vi "Actor Core.vi"(8 "error in":errorcluster, 11 "RDS Test Child in":refnum<class "RDS Test Child.lvclass">) -> (0 "error out":errorcluster, 3 "Actor out":refnum<class "Actor.lvclass">)   [LabVIEW 2015, in "RDS Test Child.lvlib" / "RDS Test Child.lvclass"]
doc: "(<B>Filename</B>: Actor Framework.lvlib:Actor.lvclass:Actor Core.vi)\n\nReceives messages to the actor, reacts to them, and initiates any error handling that may shut the actor down.\n\nDescendant classes may override this VI to append parallel tasks for the actor to complete while it handles messages. Overrides use the Call Parent Method node."
uses:
  RDS Test Child.lvclass
  RDS Parent Actor/RDS Parent Actor/RDS Parent Actor.lvclass
  <vilib>/ActorFramework/Actor/Actor.lvclass
  <vilib>/ActorFramework/Stop Msg/Stop Msg.lvclass
  Libraries/RDS Framework/RDS Message Class/RDS Message.lvclass
  Libraries/RDS Framework/RDS Message ID.ctl
  Libraries/RDS Child Messages/RDS Child Messages.lvlib
  Libraries/RDS Child Messages/String Message/String Message.lvclass
  Libraries/RDS Framework/RDS Message Class/AIP Command.lvclass
  Libraries/RDS Framework/RDS Message Class/AIP Command Control.ctl
  Libraries/RDS Child Messages/MCB/MCB Command Message/MCB Command.lvclass
  Libraries/RDS Child Messages/MCB/MCB Channel.ctl
  Libraries/3rd Party/Artificial Horizon/lv-attitudecontrol.lvlib
  Libraries/RDS Child Messages/Helm/Helm Limiter Message/Helm Limiter Msg.lvclass
  Libraries/RDS Child Messages/Helm/Heading Command/Heading Command Msg.lvclass
  Libraries/RDS Child Messages/Helm/Steering Command/Steering Command.lvclass
  Libraries/RDS Child Messages/Controller Message/Controller Message.lvclass
  Libraries/RDS Child Messages/Controller Message/Controller Message Type.ctl
  RDS Controller Actor/RDS Controller Actor/Controller.ctl
  RDS Controller Actor/RDS Controller Actor/RDS Controller Actor.lvlib
  RDS State Tracker/RDS State/RDS State.lvclass
  Libraries/RDS Child Messages/Depth Data Message/Depth Data Message.lvclass
  Libraries/RDS Child Messages/AIP Set Min Depth Message/AIP Set Min Depth Message.lvclass
  Compass Instrument/Compass Instrument.lvlib
  RDS Mission Controller Actor/RDS Mission Controller Actor.lvlib
  RDS Mission Controller Actor/MissionOp.ctl
  Libraries/RDS Child Messages/PID Gains/PID Gains Set Message.lvclass
  Libraries/RDS Instruments/AIP/AIP States.ctl
  Libraries/RDS Instruments/RDS Instrument Library.lvlib
  Libraries/RDS Instruments/AIP/AIP Status.ctl
  Libraries/3rd Party/NMEA_GPS/NMEA_LatitudeDirection.ctl
  Libraries/3rd Party/NMEA_GPS/NMEA.lvlib
  Libraries/3rd Party/NMEA_GPS/NMEA_LongitudeDirection.ctl
  Libraries/3rd Party/NMEA_GPS/NMEA_GPRMC-data.ctl
  Libraries/RDS Child Messages/MCB/MCB Motor Status.ctl
  Libraries/RDS Instruments/Compass/Compass Data.ctl
  RDS Helm Actor/RDS Helm Actor/Helm State.ctl
  RDS Helm Actor/RDS Helm Actor.lvlib
  Libraries/RDS Child Messages/Helm/Heading Command/Heading Command Cntrl.ctl
  Libraries/RDS Child Messages/Helm/Steering Command/Steering Command Cntrl.ctl
  Libraries/RDS Child Messages/PID Gains/PID Gains Control.ctl
  Libraries/RDS Child Messages/Helm/Helm Status Message/Helm Status Control.ctl
  Libraries/GUI/Throttles.ctl
  Libraries/Geo/RDS Libraries.lvlib
  Libraries/RDS Instruments/Battery/Battery Data.ctl
  Libraries/RDS Child Messages/Battery Data/Battery Status.ctl
  Libraries/RDS Child Messages/Depth Data Message/Depth Data.ctl
  RDS Mission Controller Actor/Mission Controller Navigation State.ctl
  Libraries/RDS Child Messages/Mission Messages/Mission Controller State Control.ctl
  Libraries/RDS Child Messages/Mission Messages/Mission Controller State Message.lvclass
  RDS Mission Controller Actor/Mission Controller Settings.ctl
panel:
  in  "Tab Control":T1(tab)
  out "Depth Time":timestamp
  in  "stop":bool
  out "$GPRMC Msg":T2={"TimeStamp"=timestamp(0 s since 1904-01-01), "Validity"=FALSE, "Latitude"=0.0, "Latitude-Direction"=enum."North", "Longitude"=0.0, "Longitude-Direction"=enum."East", "Speed in knots"=0.0, "True course"=0.0, "Date Stamp"=timestamp(0 s since 1904-01-01), "Magnetic Variation (East/West)"=0.0, "GPS Latitude"=0.0, "GPS Longitude"=0.0} {"GPS Longitude" format="%.6f"; "GPS Latitude" format="%.6f"; "Magnetic Variation (East/West)" format="%.02f [deg]"; "Date Stamp" format="%<%x>T"; "True course" format="%.02f [deg]"; "Speed in knots" format="%.02f [kts]"; "Longitude" format="%0.4f [long]"; "Latitude" format="%.04f [lat]"; "TimeStamp" format="%<%.2X>T"}
  in  "Port Throttle":i16
  in  "STBD Throttle":i16
  in  "Btn Port Throttle":bool
  in  "Btn STBD Throttle":bool
  out "Port Motor 2":T5
  out "STBD Motor 2":T5
  out "Compass Data":T6
  in  "Attitude Indicator":refnum<vi>(3d-picture)
  out "Depth":dbl
  out "Water Temp":dbl
  in  "btn_shutdown":bool
  in  "rckr_shutdown_safety":bool
  out "Battery Pack Time":timestamp
  out "GPS Frame Time":timestamp
  out "Compass Frame Time":timestamp
  out "Port Motor Time":timestamp
  out "STBD Motor Time":timestamp
  in  "AIP Stop":bool
  in  "AIP Stow":bool
  in  "AIP Deploy":bool
  out "AIP Status Time Stamp":timestamp
  out "AIP Status":T7
  out "Current Chart":dbl(graph)
  out "Battery Pack Info":T9
  in  "btn_gains set":bool
  in  "Gains":T11 {"D (Td)" format="%#_9f"; "I (Ti)" format="%#_9f"; "P (Kc)" format="%#.9f"}
  in  "Throttles":T12 {"STBD" scale=-1000.0..1000.0; "Port" scale=-1000.0..1000.0}
  in  "Steering Command":T13
  in  "Heading Command":T14
  in  "btn_limiter_set":bool
  in  "Limter":dbl(slide) min=0.0 max=100.0 scale=0.0..100.0
  out "Helm Status":T15 {"Gains"."D (Td)" format="%#_9f"; "Gains"."I (Ti)" format="%#_9f"; "Gains"."P (Kc)" format="%#.9f"}
  out "Rudder Chart":dbl(graph)
  out "PV and S Chart":cluster{"initial PV":dbl, "SP:":dbl}(graph)
  out "Helm Status Time":timestamp
  in  "btn_heading_command":bool
  in  "btn_steering_command":bool
  out "Message time":dbl
  in  "btn_set_mag_dev":bool
  in  "Compass Mag Dev":dbl
  in  "btn_set_aip_min_depth":bool
  in  "AIP Min Depth":dbl
  in  "btn_sim_depth_data":bool
  in  "Depth Data":T17
  in  "btn_shore_remote_ReqControl":bool
  in  "btn_shore_remote_Relinquish":bool
  in  "btn_local_remote_Relinquish":bool
  in  "btn_local_remote_ReqControl":bool
  in  "Send Msg":bool
  out "String":string
  in  "Send string":bool
  in  "String 2":string
  in  "btn_open_mission":bool
  in  "btn_save_mission":bool
  out "XY Graph":T18(graph)
  in  "btn_send settings":bool
  in  "btn_set_op_run":bool
  in  "btn_upload_mission":bool
  in  "Test Mission":T19[](array[typedef]) {"GPS Longitude" format="%.6g"; "GPS Latitude" format="%.6g"}
  out "Mission Controller State":T20 {"Mission"."GPS Longitude" format="%.6g"; "Mission"."GPS Latitude" format="%.6g"}
  in  "btn_mission_Relinquish":bool
  in  "btn_mission_ReqControl":bool
  in  "Mission Controller Settings":T22
  in  "MissionOp Index":i32
  in  "RDS State":refnum<class "RDS State.lvclass">
  out "State Sample Time":timestamp
  out "Controller State":T23
  out "Helm Status 2":T15 {"Gains"."D (Td)" format="%#_9f"; "Gains"."I (Ti)" format="%#_9f"; "Gains"."P (Kc)" format="%#.9f"}
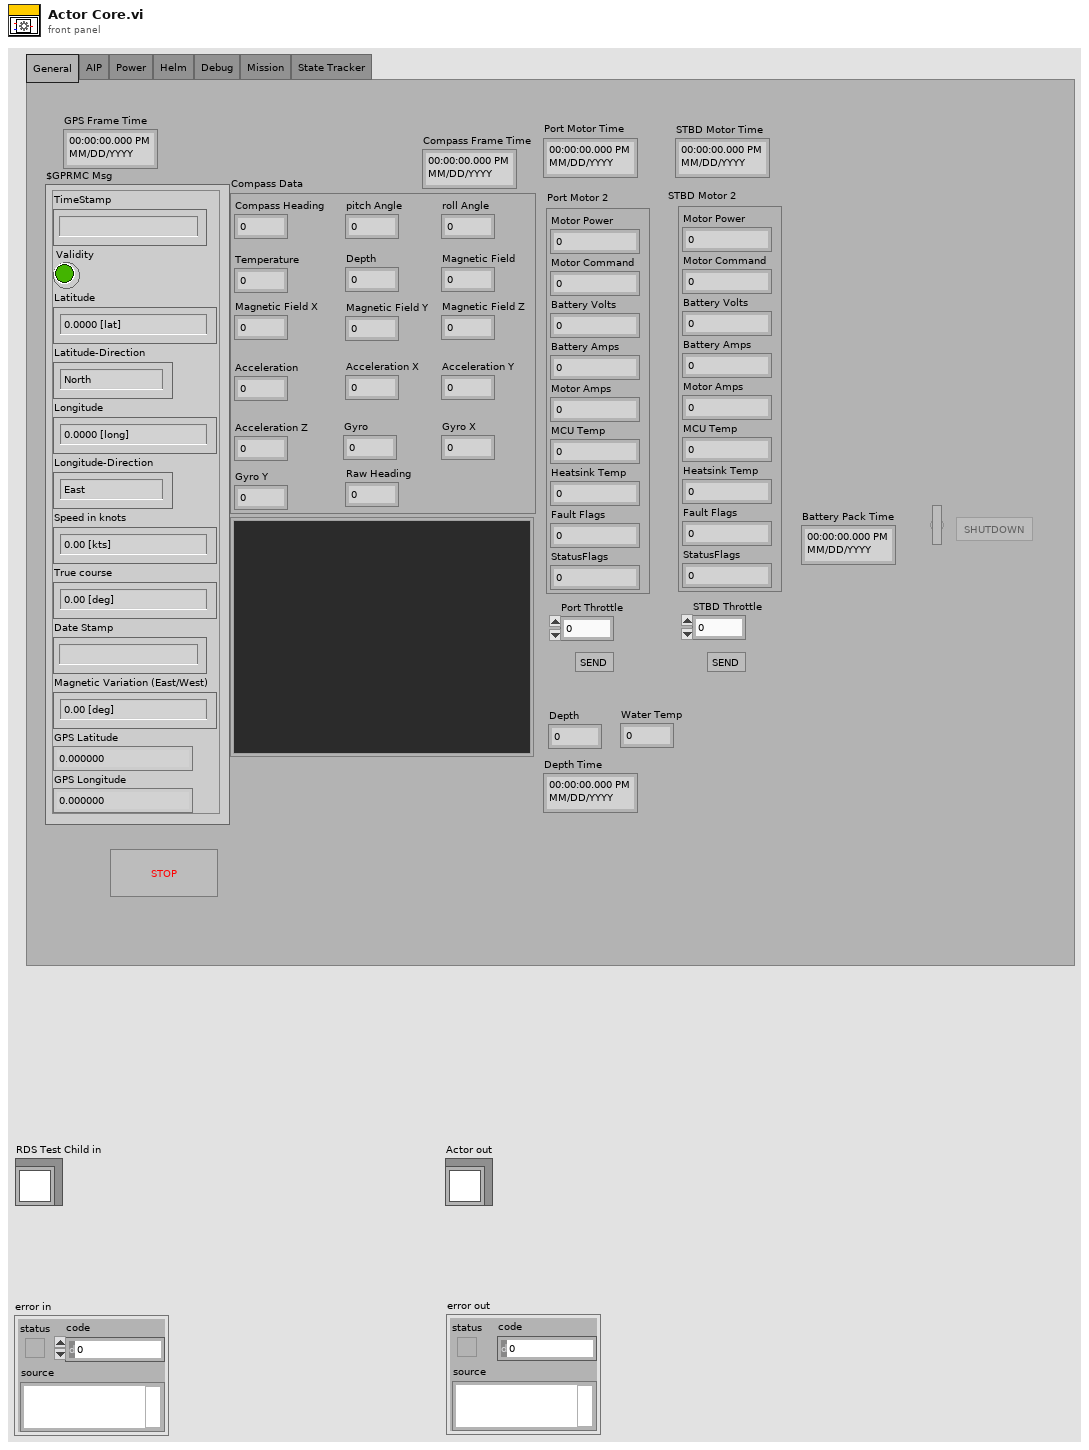
[diagram p1: front panel]
types:
  T1 = enum32{"General", "AIP", "Power", "Helm", "Debug", "Mission", "State Tracker"}
  T2 = typedef "RDS Libraries.lvlib/NMEA.lvlib/NMEA_GPRMC-data.ctl" = cluster{"TimeStamp":timestamp, "Validity":bool, "Latitude":dbl, "Latitude-Direction":T3, "Longitude":dbl, "Longitude-Direction":T4, "Speed in knots":sgl, "True course":sgl, "Date Stamp":timestamp, "Magnetic Variation (East/West)":sgl, "GPS Latitude":dbl, "GPS Longitude":dbl}
  T3 = typedef "RDS Libraries.lvlib/NMEA.lvlib/NMEA_LatitudeDirection.ctl" = enum16{"", "North", "South"}
  T4 = typedef "RDS Libraries.lvlib/NMEA.lvlib/NMEA_LongitudeDirection.ctl" = enum16{"", "East", "West"}
  T5 = typedef "RDS Child Messages.lvlib/MCB Motor Status.ctl" = cluster{"Motor Power":i16, "Motor Command":i16, "Battery Volts":sgl, "Battery Amps":sgl, "Motor Amps":sgl, "MCU Temp":i16, "Heatsink Temp":i16, "Fault Flags":u16, "StatusFlags":u16}
  T6 = typedef "RDS Instrument Library.lvlib/Compass Data.ctl" = cluster{"Compass Heading":sgl, "pitch Angle":sgl, "roll Angle":sgl, "Temperature":sgl, "Depth":sgl, "Magnetic Field":sgl, "Magnetic Field X":sgl, "Magnetic Field Y":sgl, "Magnetic Field Z":sgl, "Acceleration":sgl, "Acceleration X":sgl, "Acceleration Y":sgl, "Gyro":sgl, "Gyro X":sgl, "Acceleration Z":sgl, "Gyro Y":sgl, "Raw Heading":sgl}
  T7 = typedef "RDS Instrument Library.lvlib/AIP Status.ctl" = cluster{"FWD Port":T8, "FWD Stbd":T8, "AFT Port":T8, "AFT Stbd":T8, "AIP Depth Min":u8}
  T8 = typedef "RDS Instrument Library.lvlib/AIP States.ctl" = enum16{"Deploy", "Deploying", "Deployed", "Stow", "Stowing", "Stowed", "Fault", "brakeOnStow", "breakOnDeploy", "Stopped", "Stopping"}
  T9 = typedef "RDS Instrument Library.lvlib/Battery Data.ctl" = cluster{"Battery Status":T10, "Pack Voltage":sgl, "Pack Current":sgl, "Pack Capacity":sgl, "Max Cell Temp":sgl, "Min Cell Temp":sgl, "Max Cell Voltage":sgl, "Min Cell Voltage":sgl}
  T10 = typedef "RDS Instrument Library.lvlib/Battery Status.ctl" = enum16{"Pack Normal", "Alarm: Cell temp too high", "Alarm: Pack voltage too high", "Warn: Pack voltage too high ", "Alarm: Pack voltage too low", "Warn: Pack voltage low", "Alarm Pack current too high", "Warn: Pack current too high ", "Fault: Pack to chassis connection detected", "Fault: Pack to cell connection error", "Fautl: System error"}
  T11 = typedef "RDS Child Messages.lvlib/PID Gains Control.ctl" = cluster{"P (Kc)":sgl, "I (Ti)":sgl, "D (Td)":sgl}
  T12 = typedef "RDS Libraries.lvlib/Throttles.ctl" = cluster{"Port":dbl, "STBD":dbl}
  T13 = typedef "RDS Child Messages.lvlib/Steering Command Cntrl.ctl" = cluster{"Throttle":i16, "Rudder":i8, "Duration (s)":u16}
  T14 = typedef "RDS Child Messages.lvlib/Heading Command Cntrl.ctl" = cluster{"Throttle":i16, "Heading":sgl, "Duration (s)":i16}
  T15 = typedef "RDS Child Messages.lvlib/Helm Status Control.ctl" = cluster{"Helm State":T16, "Heading Command Control":T14, "Steering Command Control":T13, "Last Command Time":timestamp, "Gains":T11, "Current Heading":dbl, "Port Throttle":i16, "STBD Throttle":i16, "Limiter":dbl}
  T16 = typedef "RDS Helm Actor.lvlib/Helm State.ctl" = enum16{"Idle", "Executing Heading Command", "Executing Steering Command"}
  T17 = typedef "RDS Child Messages.lvlib/Depth Data.ctl" = cluster{"Depth":sgl, "Water Temp":i8}
  T18 = cluster{"GPS Latitude":ext, "GPS Longitude":ext}[]
  T19 = typedef "RDS Mission Controller Actor.lvlib/MissionOp.ctl" = cluster{"MissionOp Type":enum16{"Waypoint", "Loiter", "Wait", "Deploy AIP", "Stow AIP"}, "Duration (s)":u16, "Throttle":i16, "GPS Latitude":dbl, "GPS Longitude":dbl, "Loiter Range (m)":u16}
  T20 = typedef "RDS Child Messages.lvlib/Mission Controller State Message.lvclass/Mission Controller State Control.ctl" = cluster{"iHasControl":bool, "controlTimer":timestamp, "Nav State":T21, "Current MissionOp Index":i32, "Mission":T19[], "Distance to Target":dbl, "Seconds to Timeout":dbl}
  T21 = typedef "RDS Mission Controller Actor.lvlib/Mission Controller Navigation State.ctl" = cluster{"GPS Latitude":ext, "GPS Longitude":ext, "Compass Heading":dbl, "Speed":dbl}
  T22 = typedef "RDS Mission Controller Actor.lvlib/Mission Controller Settings.ctl" = cluster{"Waypoint Radius (m)":dbl}
  T23 = typedef "RDS Controller Actor.lvlib/Controller.ctl" = enum16{"Idle", "Local Remote Control", "Shore Remote Control", "Mission Control"}
  T24 = enum8{"Enabled", "Disabled", "Disabled and Grayed Out"}
  T25 = typedef "RDS Libraries.lvlib/lv-attitudecontrol.lvlib/AttitudeHandle.ctl" = cluster{"First Scene Object":refnum<vi>, "Drum":refnum<vi>, "Window":refnum<vi>, "Dial":refnum<vi>, "Scene Graph":refnum<vi>, "Last Drum Pitch":dbl, "Last Drum Roll ":dbl, "Last Dial Roll":dbl}
  T26 = typedef "RDS Child Messages.lvlib/RDS Message ID.ctl" = enum16{"RDS Hello World", "String Message", "AIP_Status", "AIP_Command", "GPS_Data", "MCB_Command", "MCB_Status", "Compass_Data", "Depth_Data", "Battery_Data", "Contoller_State", "Set_Mag_Dev", "BTB_Shutdown", "State_Sample_Request", "State_Sample", "PID_Gains_Set", "Helm_Limiter_Set", "Helm_Heading_Command", "Helm_Steering_Command", "Helm_Status", "Controller_Message", "AIP_Set_Min_Depth", "Mission_Controller_State", "Mission_Upload", "Mission_Set_Op_and_Run", "Mission_Settings_Set"}
  T27 = typedef "RDS Child Messages.lvlib/AIP Command Control.ctl" = enum16{"Stow", "Deploy", "Stop", "Validate Sensors", "Jog Deploy FP", "Jog Stow FP", "Jog Deploy FS", "Jog Stow FS", "Jog Deploy AP", "Jog Stow AP", "Jog Deploy AS", "Jog Stow AS", "Deploy FP", "Deploy FS", "Deploy AP", "Deploy AS", "Stow FP", "Stow FS", "Stow AP", "Stow AS"}
  T28 = typedef "RDS Child Messages.lvlib/MCB Channel.ctl" = enum16{"PORT", "STBD"}
  T29 = typedef "RDS Child Messages.lvlib/Controller Message.lvclass/Controller Message Type.ctl" = enum16{"Control Relinquish Request", "Control Relinquish Command", "Control Request", "Control Granted"}
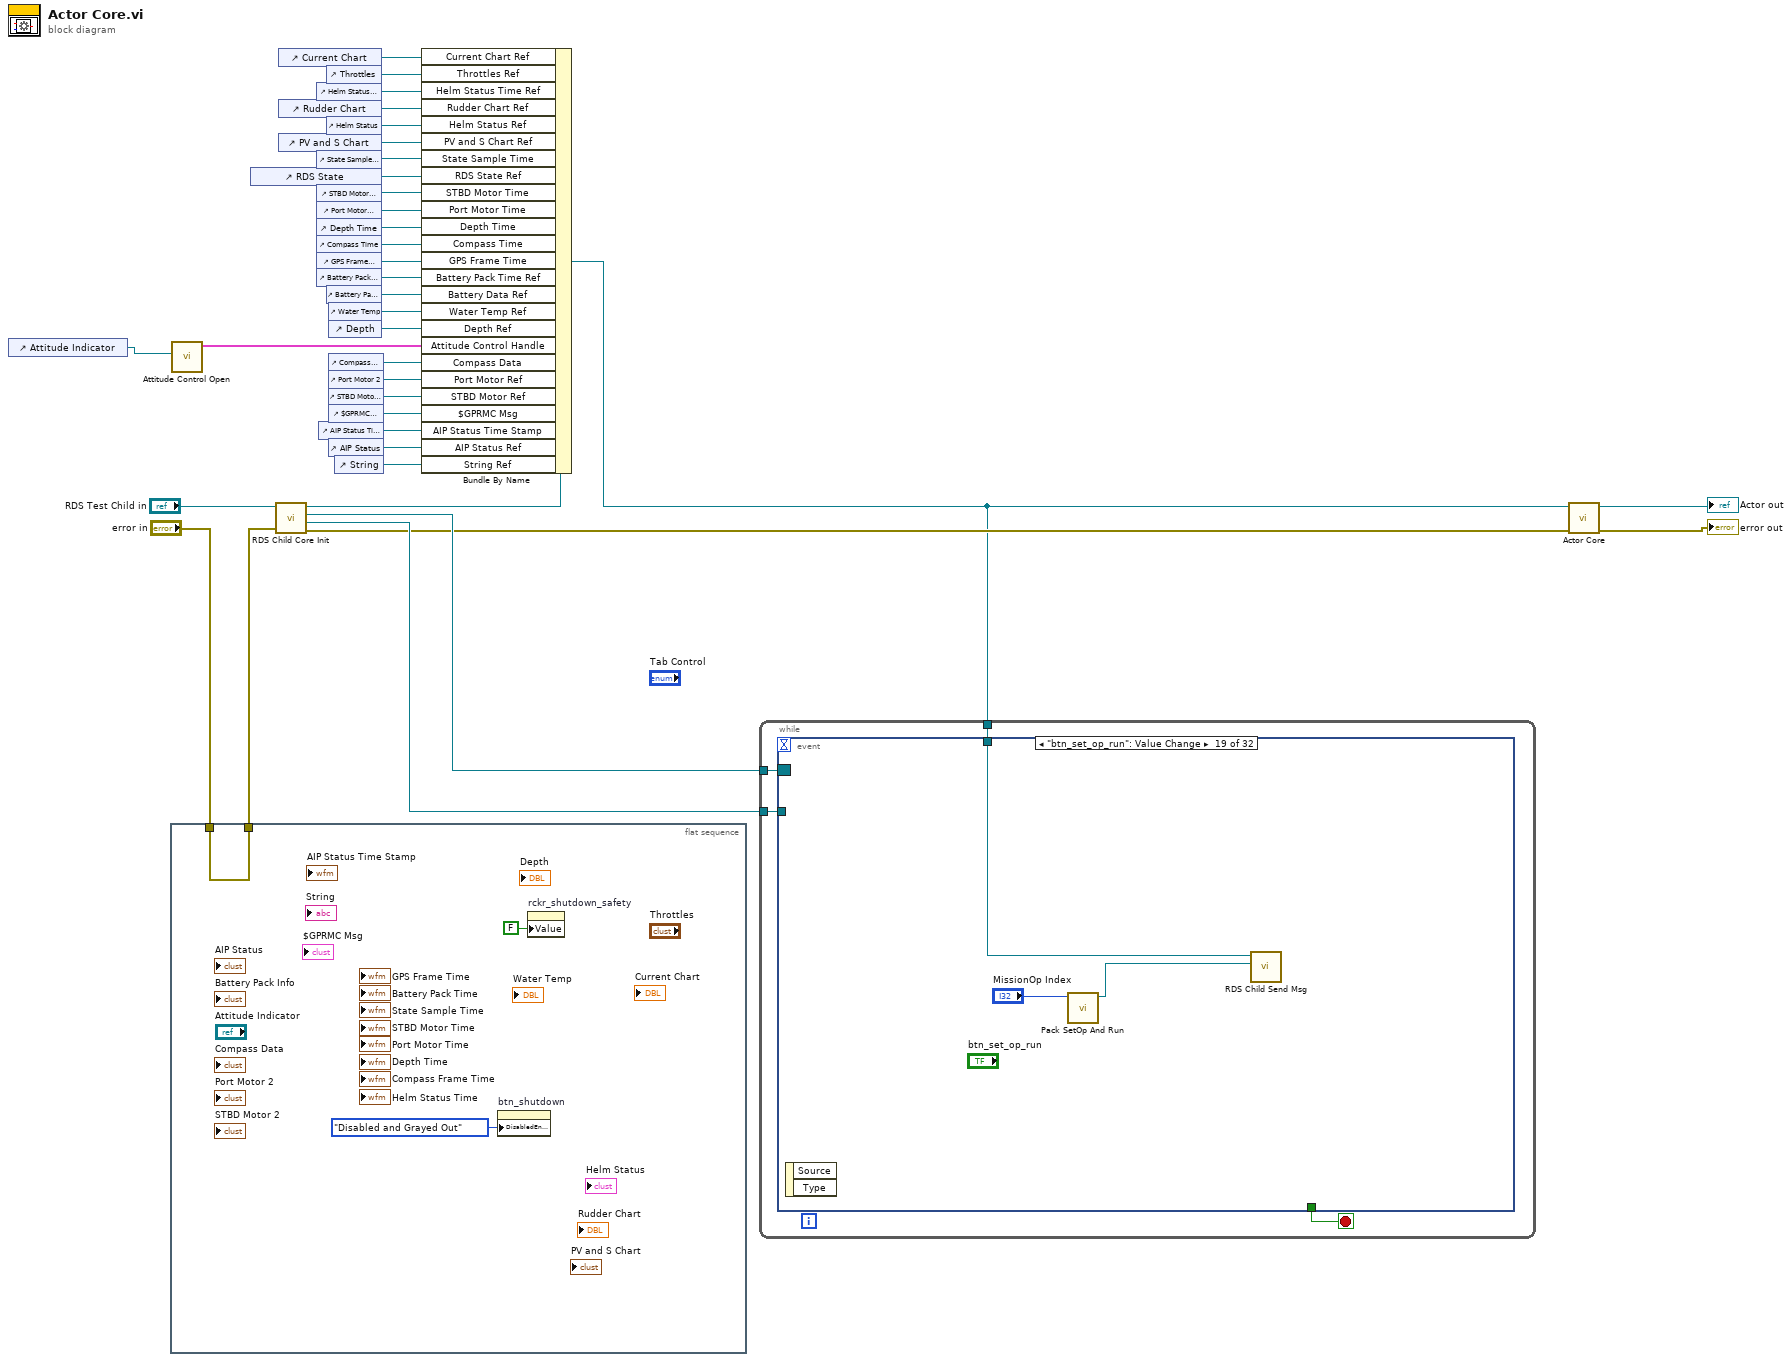
[diagram p0: block diagram]
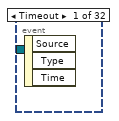
[diagram p2: hidden frame]
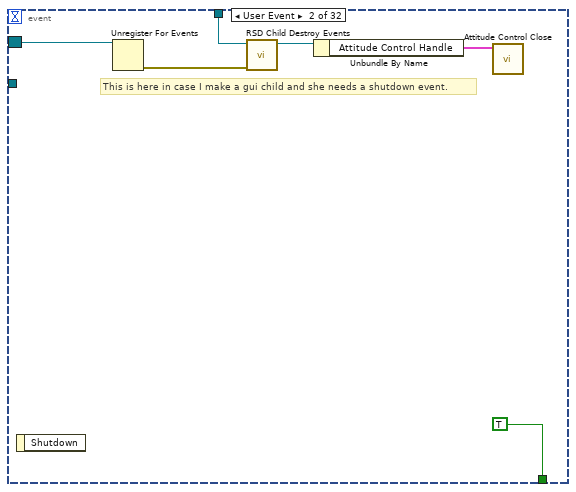
[diagram p3: hidden frame]
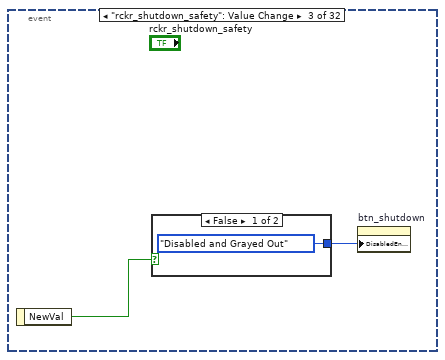
[diagram p4: hidden frame]
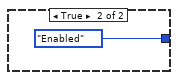
[diagram p5: hidden frame]
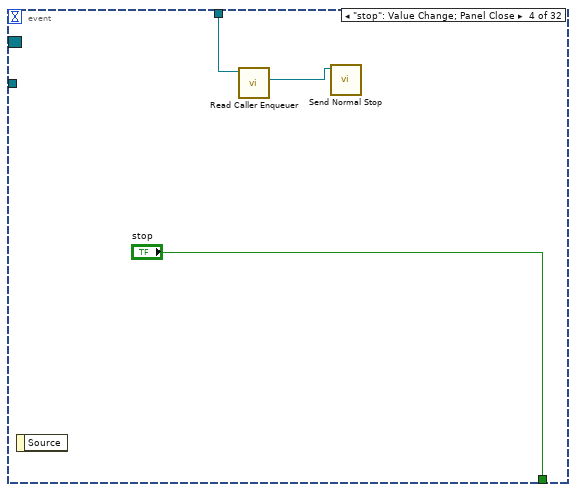
[diagram p6: hidden frame]
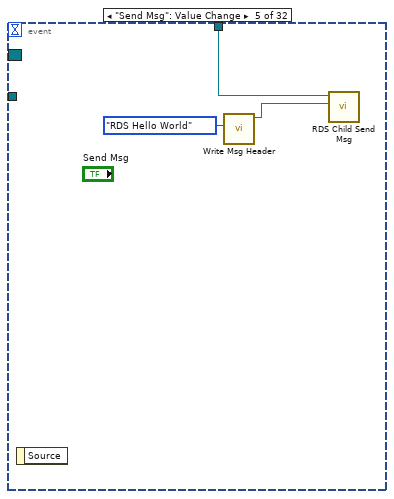
[diagram p7: hidden frame]
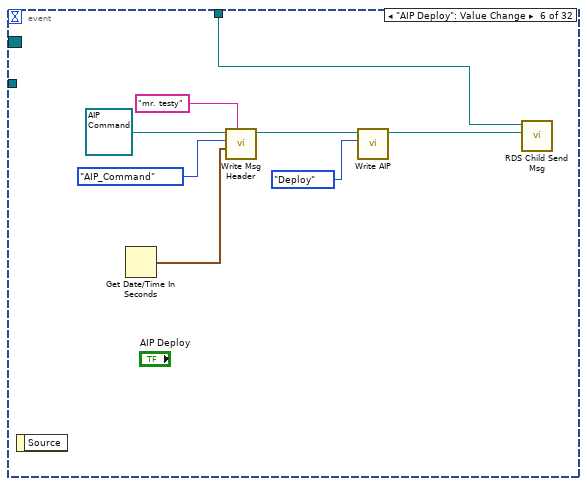
[diagram p8: hidden frame]
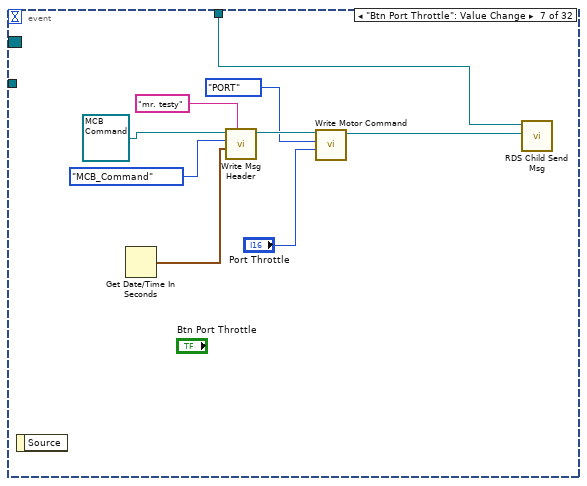
[diagram p9: hidden frame]
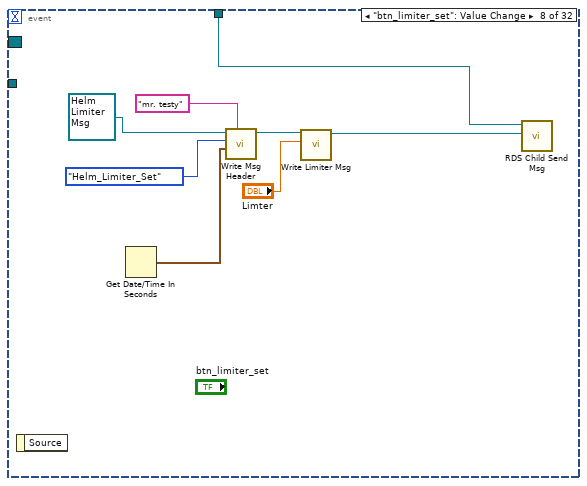
[diagram p10: hidden frame]
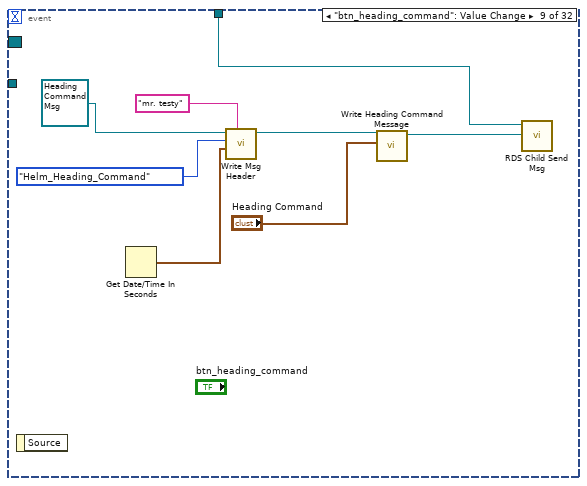
[diagram p11: hidden frame]
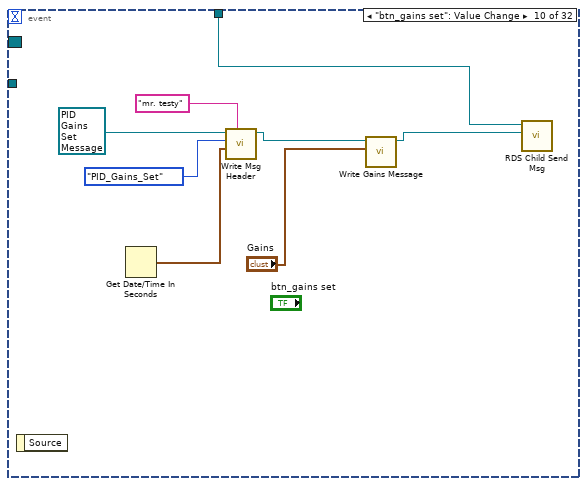
[diagram p12: hidden frame]
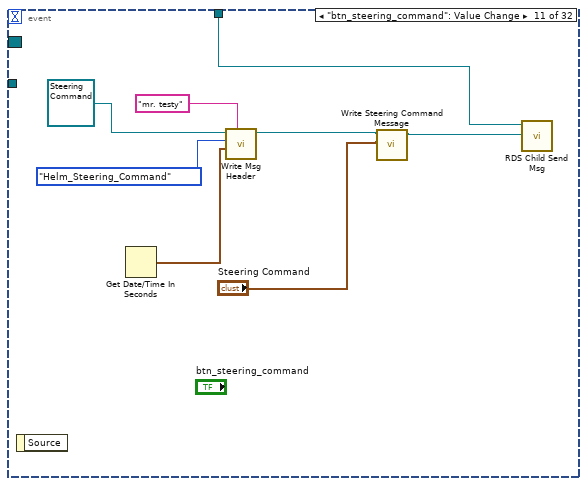
[diagram p13: hidden frame]
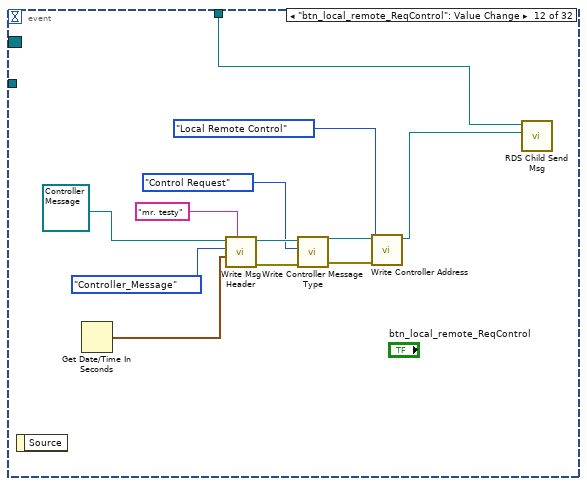
[diagram p14: hidden frame]
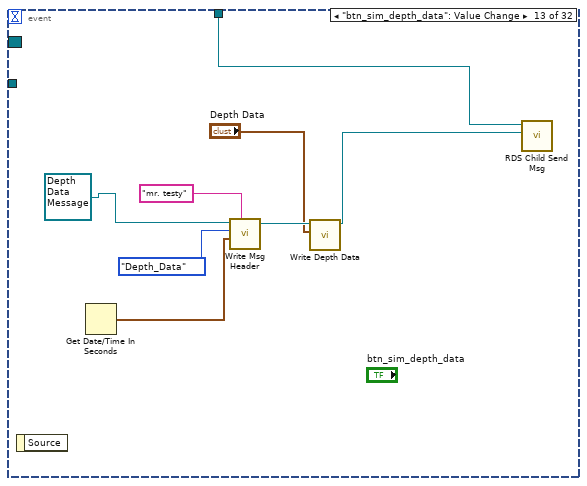
[diagram p15: hidden frame]
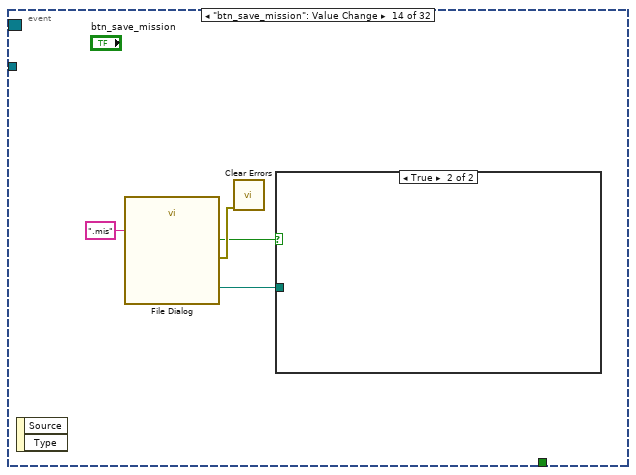
[diagram p16: hidden frame]
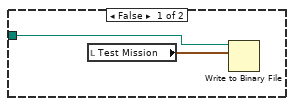
[diagram p17: hidden frame]
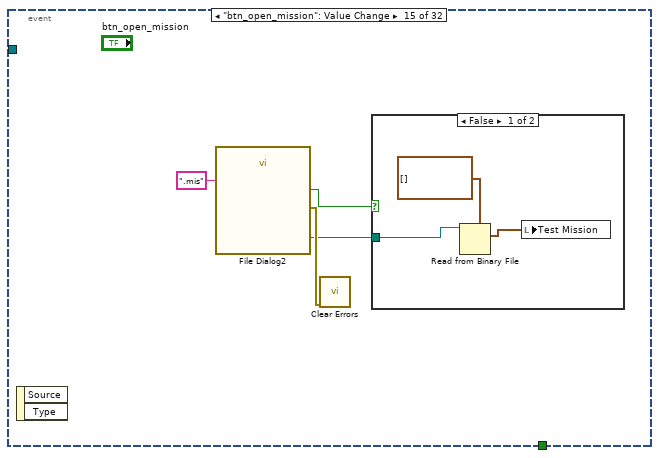
[diagram p18: hidden frame]
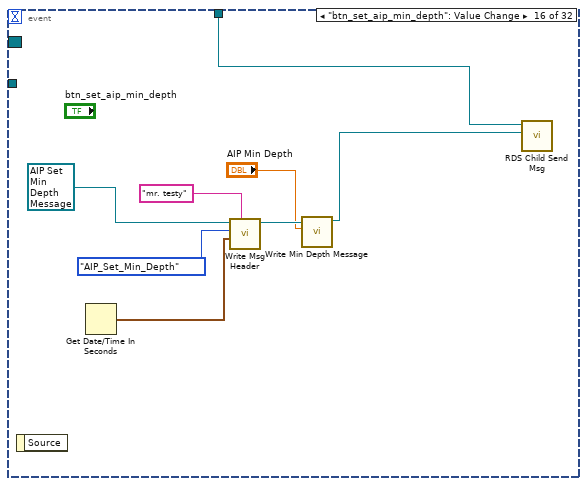
[diagram p20: hidden frame]
diagram:
  n1 = control-ref of="Attitude Indicator"() -> (w21:refnum<vi>)
  n2 = flat-sequence {
    tunnel: [w39] -> w16
    tunnel: "error in" -> [w39]
    frame #0 {
      n3 = property on="btn_shutdown" class="Bool"("DisabledEnum"=T24."Disabled and Grayed Out" ("Disabled")) -> ()  [unwired: 2 in, 2 out]
      n4 = property on="rckr_shutdown_safety" class="Bool (strict)"("Value"=FALSE ("rckr_shutdown_safety")) -> ()  [unwired: 2 in, 2 out]
    }
  }
  n5 = call "Attitude Control Open.vi"("Scene Graph"=w21) -> ("Attitude Control Handle"=w20:T25)  [unwired: 9 in, 1 out]
  n6 = control-ref of="RDS State"() -> (w7:refnum<vi>)
  n7 = call "RDS Child Core Init.vi"("error in (no error)"=w16, "RDS Parent Actor in"="RDS Test Child in") -> ("error out"=w33:errorcluster, "RDS Router Enqeuer"=w34:refnum<class "Message Enqueuer.lvclass">, "Event Registration Refnum"=w35:refnum<event-registration>, "RDS Parent Actor out"=w30:refnum<class "RDS Test Child.lvclass">)  [unwired: 6 in]
  n8 = control-ref of="Current Chart"() -> (w1:refnum<vi>)
  n9 = control-ref of="Rudder Chart"() -> (w4:refnum<vi>)
  n10 = control-ref of="PV and S Chart"() -> (w6:refnum<vi>)
  n11 = control-ref of="Helm Status Time"() -> (w3:refnum<vi>)
  n12 = control-ref of="State Sample Time"() -> (w8:refnum<vi>)
  n13 = control-ref of="STBD Motor Time"() -> (w9:refnum<vi>)
  n14 = control-ref of="Port Motor Time"() -> (w10:refnum<vi>)
  n15 = control-ref of="Depth Time"() -> (w11:refnum<vi>)
  n16 = control-ref of="Compass Time"() -> (w12:refnum<vi>)
  n17 = control-ref of="GPS Frame Time"() -> (w13:refnum<vi>)
  n18 = control-ref of="Battery Pack Time"() -> (w14:refnum<vi>)
  n19 = control-ref of="AIP Status Time Stamp"() -> (w26:refnum<vi>)
  n20 = control-ref of="Throttles"() -> (w2:refnum<vi>)
  n21 = control-ref of="Helm Status"() -> (w5:refnum<vi>)
  n22 = control-ref of="Battery Pack Info"() -> (w15:refnum<vi>)
  n23 = control-ref of="Water Temp"() -> (w19:refnum<vi>)
  n24 = control-ref of="Depth"() -> (w18:refnum<vi>)
  n25 = control-ref of="Compass Data"() -> (w22:refnum<vi>)
  n26 = control-ref of="Port Motor 2"() -> (w24:refnum<vi>)
  n27 = control-ref of="STBD Motor 2"() -> (w23:refnum<vi>)
  n28 = control-ref of="$GPRMC Msg"() -> (w25:refnum<vi>)
  n29 = control-ref of="AIP Status"() -> (w27:refnum<vi>)
  n30 = control-ref of="String"() -> (w28:refnum<vi>)
  n31 = Bundle By Name(cluster=w30, "Current Chart Ref"=w1, "Throttles Ref"=w2, "Helm Status Time Ref"=w3, "Rudder Chart Ref"=w4, "Helm Status Ref"=w5, "PV and S Chart Ref"=w6, "State Sample Time"=w8, "RDS State Ref"=w7, "STBD Motor Time"=w9, "Port Motor Time"=w10, "Depth Time"=w11, "Compass Time"=w12, "GPS Frame Time"=w13, "Battery Pack Time Ref"=w14, "Battery Data Ref"=w15, "Water Temp Ref"=w19, "Depth Ref"=w18, "Attitude Control Handle"=w20, "Compass Data"=w22, "Port Motor Ref"=w24, "STBD Motor Ref"=w23, "$GPRMC Msg"=w25, "AIP Status Time Stamp"=w26, "AIP Status Ref"=w27, "String Ref"=w28) -> (w29:refnum<class "RDS Test Child.lvclass">)
  n32 = while {
    tunnel: w35 -> [w43]
    tunnel: w29 -> [w41]
    tunnel: w34 -> [w40]
    stop <- w42 stop-if-true
    n33 = event shown="[18] \"btn_set_op_run\": Value Change" {
      selector: w43 -> [_ w48 _ _ _ _ _ _ _ _ _ _ _ _ _ _ _ _ _ _ _ _ _ _ _ _ _ _ _ _ _ _]
      dyn-events: _ -> [_ _ _ _ _ _ _ _ _ _ _ _ _ _ _ _ _ _ _ _ _ _ _ _ _ _ _ _ _ _ _ _]
      timeout: _ -> [_ _ _ _ _ _ _ _ _ _ _ _ _ _ _ _ _ _ _ _ _ _ _ _ _ _ _ _ _ _ _ _]
      tunnel: [_ TRUE _ "stop" _ _ _ _ _ _ _ _ _ _ _ _ _ _ _ _ _ _ _ _ _ _ _ _ _ _ _ _] -> w42
      tunnel: w41 -> [_ w47 _ w56 w59 w60 w73 w81 w89 w97 w105 w117 w125 _ _ w146 w152 w155 w157 w160 _ w184 w196 w208 w220 w232 _ w244 w248 w256 w266 w278]
      tunnel: w40 -> [_ _ _ _ _ _ _ _ _ _ _ _ _ _ _ _ _ _ _ _ _ _ _ _ _ _ _ _ _ _ _ _]
      event Timeout {
        n34 = event-data() -> ()  [unwired: 1 in, 3 out]
      }
      event User Event {
        # "This is here in case I make a gui child and she needs a shutdown event."
        n35 = event-data() -> ()  [unwired: 1 in, 1 out]
        n36 = Unregister For Events(event registration refnum=w48) -> (error out=w46:errorcluster)  [unwired: 1 in]
        n37 = call "RSD Child Destroy Events.vi"("error in (no error)"=w46, "RDS Parent Actor in"=w47) -> ("RDS Parent Actor out"=w45:refnum<class "RDS Test Child.lvclass">)  [unwired: 8 in, 1 out]
        n38 = Unbundle By Name(w45) -> ("Attitude Control Handle"=w44:T25)
        n39 = call "Attitude Control Close.vi"("Attitude Control Handle"=w44) -> ()  [unwired: 10 in, 1 out]
      }
      event "rckr_shutdown_safety": Value Change {
        n40 = event-data() -> ("NewVal"=w51:bool)  [unwired: 1 in]
        n41 = case shown="False" w51 {
          tunnel: [T24."Disabled and Grayed Out" ("Disabled") T24."Enabled" ("Disabled")] -> w50
          frame False {
          }
          frame True {
          }
        }
        n42 = property on="btn_shutdown" class="Bool"("DisabledEnum"=w50) -> ()  [unwired: 2 in, 2 out]
      }
      event "stop": Value Change; Panel Close {
        n43 = event-data() -> ()  [unwired: 1 in, 1 out]
        n44 = call <vilib>:"Read Caller Enqueuer.vi"("Actor"=w56) -> ("Caller Enqueuer"=w55:refnum<class "Message Enqueuer.lvclass">)  [unwired: 10 in]
        n45 = call <vilib>:"Send Normal Stop.vi"("Message Enqueuer"=w55) -> ()  [unwired: 10 in, 1 out]
      }
      event "Send Msg": Value Change {
        n46 = event-data() -> ()  [unwired: 1 in, 1 out]
        n47 = call "Write Msg Header.vi"("Msg ID"=RDS_Message_ID."RDS Hello World") -> ("RDS Message out"=w57:refnum<class "RDS Message.lvclass">)  [unwired: 9 in, 1 out]
        n48 = call "RDS Child Send Msg.vi"("RDS Message"=w57, "RDS Parent Actor in"=w59) -> ()  [unwired: 8 in, 2 out]
      }
      event "AIP Deploy": Value Change {
        n49 = event-data() -> ()  [unwired: 1 in, 1 out]
        n50 = Get Date/Time In Seconds() -> (seconds since 1Jan1904=w64:timestamp)
        n51 = call "Write Msg Header.vi"("Sender Name"="mr. testy", "Time Stamp"=w64, "Msg ID"=RDS_Message_ID."AIP_Command", "RDS Message in"=refnum<class "AIP Command.lvclass"> refnum ("RDS Child Messages.lvlib:AIP Command.lvclass")) -> ("RDS Message out"=w65:refnum<class "AIP Command.lvclass">)  [unwired: 6 in, 1 out]
        n52 = call "Write AIP.vi"("AIP Command"=AIP_Command_Control."Deploy", "AIP Deploy Command in"=w65) -> ("AIP Deploy Command out"=w61:refnum<class "AIP Command.lvclass">)  [unwired: 8 in, 1 out]
        n53 = call "RDS Child Send Msg.vi"("RDS Message"=w61, "RDS Parent Actor in"=w60) -> ()  [unwired: 8 in, 2 out]
      }
      event "Btn Port Throttle": Value Change {
        n54 = event-data() -> ()  [unwired: 1 in, 1 out]
        n55 = Get Date/Time In Seconds() -> (seconds since 1Jan1904=w75:timestamp)
        n56 = call "Write Msg Header.vi"("Sender Name"="mr. testy", "Time Stamp"=w75, "Msg ID"=RDS_Message_ID."MCB_Command", "RDS Message in"=refnum<class "MCB Command.lvclass"> refnum ("RDS Child Messages.lvlib:MCB Command.lvclass")) -> ("RDS Message out"=w71:refnum<class "MCB Command.lvclass">)  [unwired: 6 in, 1 out]
        n57 = call "Write Motor Command.vi"("Motor Command"="Port Throttle", "Motor"=MCB_Channel."PORT", "MCB Command in"=w71) -> ("MCB Command out"=w68:refnum<class "MCB Command.lvclass">)  [unwired: 7 in, 1 out]
        n58 = call "RDS Child Send Msg.vi"("RDS Message"=w68, "RDS Parent Actor in"=w73) -> ()  [unwired: 8 in, 2 out]
      }
      event "btn_limiter_set": Value Change {
        n59 = event-data() -> ()  [unwired: 1 in, 1 out]
        n60 = Get Date/Time In Seconds() -> (seconds since 1Jan1904=w83:timestamp)
        n61 = call "Write Msg Header.vi"("Sender Name"="mr. testy", "Time Stamp"=w83, "Msg ID"=RDS_Message_ID."Helm_Limiter_Set", "RDS Message in"=refnum<class "Helm Limiter Msg.lvclass"> refnum ("RDS Child Messages.lvlib:Helm Limiter Msg.lvclass")) -> ("RDS Message out"=w79:refnum<class "Helm Limiter Msg.lvclass">)  [unwired: 6 in, 1 out]
        n62 = call "Write Limiter Msg.vi"("Limiter"="Limter", "Helm Limiter Msg in"=w79) -> ("Helm Limiter Msg out"=w78:refnum<class "Helm Limiter Msg.lvclass">)  [unwired: 8 in, 1 out]
        n63 = call "RDS Child Send Msg.vi"("RDS Message"=w78, "RDS Parent Actor in"=w81) -> ()  [unwired: 8 in, 2 out]
      }
      event "btn_heading_command": Value Change {
        n64 = event-data() -> ()  [unwired: 1 in, 1 out]
        n65 = Get Date/Time In Seconds() -> (seconds since 1Jan1904=w91:timestamp)
        n66 = call "Write Msg Header.vi"("Sender Name"="mr. testy", "Time Stamp"=w91, "Msg ID"=RDS_Message_ID."Helm_Heading_Command", "RDS Message in"=refnum<class "Heading Command Msg.lvclass"> refnum ("RDS Child Messages.lvlib:Heading Command Msg.lvclass")) -> ("RDS Message out"=w87:refnum<class "Heading Command Msg.lvclass">)  [unwired: 6 in, 1 out]
        n67 = call "Write Heading Command Message.vi"("Heading Command Control"="Heading Command", "Heading Command Msg in"=w87) -> ("Heading Command Msg out"=w86:refnum<class "Heading Command Msg.lvclass">)  [unwired: 8 in, 1 out]
        n68 = call "RDS Child Send Msg.vi"("RDS Message"=w86, "RDS Parent Actor in"=w89) -> ()  [unwired: 8 in, 2 out]
      }
      event "btn_gains set": Value Change {
        n69 = event-data() -> ()  [unwired: 1 in, 1 out]
        n70 = Get Date/Time In Seconds() -> (seconds since 1Jan1904=w99:timestamp)
        n71 = call "Write Msg Header.vi"("Sender Name"="mr. testy", "Time Stamp"=w99, "Msg ID"=RDS_Message_ID."PID_Gains_Set", "RDS Message in"=refnum<class "PID Gains Set Message.lvclass"> refnum ("RDS Child Messages.lvlib:PID Gains Set Message.lvclass")) -> ("RDS Message out"=w95:refnum<class "PID Gains Set Message.lvclass">)  [unwired: 6 in, 1 out]
        n72 = call "Write Gains Message.vi"("Gains"="Gains", "PID Gains Set Message in"=w95) -> ("PID Gains Set Message out"=w93:refnum<class "PID Gains Set Message.lvclass">)  [unwired: 8 in, 1 out]
        n73 = call "RDS Child Send Msg.vi"("RDS Message"=w93, "RDS Parent Actor in"=w97) -> ()  [unwired: 8 in, 2 out]
      }
      event "btn_steering_command": Value Change {
        n74 = event-data() -> ()  [unwired: 1 in, 1 out]
        n75 = Get Date/Time In Seconds() -> (seconds since 1Jan1904=w107:timestamp)
        n76 = call "Write Msg Header.vi"("Sender Name"="mr. testy", "Time Stamp"=w107, "Msg ID"=RDS_Message_ID."Helm_Steering_Command", "RDS Message in"=refnum<class "Steering Command.lvclass"> refnum ("RDS Child Messages.lvlib:Steering Command.lvclass")) -> ("RDS Message out"=w103:refnum<class "Steering Command.lvclass">)  [unwired: 6 in, 1 out]
        n77 = call "Write Steering Command Message.vi"("Steering Command Control"="Steering Command", "Steering Command in"=w103) -> ("Steering Command out"=w104:refnum<class "Steering Command.lvclass">)  [unwired: 8 in, 1 out]
        n78 = call "RDS Child Send Msg.vi"("RDS Message"=w104, "RDS Parent Actor in"=w105) -> ()  [unwired: 8 in, 2 out]
      }
      event "btn_local_remote_ReqControl": Value Change {
        n79 = event-data() -> ()  [unwired: 1 in, 1 out]
        n80 = Get Date/Time In Seconds() -> (seconds since 1Jan1904=w119:timestamp)
        n81 = call "Write Msg Header.vi"("Sender Name"="mr. testy", "Time Stamp"=w119, "Msg ID"=RDS_Message_ID."Controller_Message", "RDS Message in"=refnum<class "Controller Message.lvclass"> refnum ("RDS Child Messages.lvlib:Controller Message.lvclass")) -> ("error out"=w115:errorcluster, "RDS Message out"=w114:refnum<class "Controller Message.lvclass">)  [unwired: 6 in]
        n82 = call "Write Controller Message Type.vi"("error in (no error)"=w115, "Controller Message Type"=Controller_Message_Type."Control Request", "Controller Message in"=w114) -> ("error out"=w111:errorcluster, "Controller Message out"=w112:refnum<class "Controller Message.lvclass">)  [unwired: 7 in]
        n83 = call "Write Controller Address.vi"("error in (no error)"=w111, "Controller"=Controller."Local Remote Control", "Controller Message in"=w112) -> ("Controller Message out"=w110:refnum<class "Controller Message.lvclass">)  [unwired: 7 in, 1 out]
        n84 = call "RDS Child Send Msg.vi"("RDS Message"=w110, "RDS Parent Actor in"=w117) -> ()  [unwired: 8 in, 2 out]
      }
      event "btn_sim_depth_data": Value Change {
        n85 = event-data() -> ()  [unwired: 1 in, 1 out]
        n86 = Get Date/Time In Seconds() -> (seconds since 1Jan1904=w127:timestamp)
        n87 = call "Write Msg Header.vi"("Sender Name"="mr. testy", "Time Stamp"=w127, "Msg ID"=RDS_Message_ID."Depth_Data", "RDS Message in"=refnum<class "Depth Data Message.lvclass"> refnum ("RDS Child Messages.lvlib:Depth Data Message.lvclass")) -> ("RDS Message out"=w123:refnum<class "Depth Data Message.lvclass">)  [unwired: 6 in, 1 out]
        n88 = call "Write Depth Data.vi"("Depth Data"="Depth Data", "Depth Data Message in"=w123) -> ("Depth Data Message out"=w121:refnum<class "Depth Data Message.lvclass">)  [unwired: 8 in, 1 out]
        n89 = call "RDS Child Send Msg.vi"("RDS Message"=w121, "RDS Parent Actor in"=w125) -> ()  [unwired: 8 in, 2 out]
      }
      event "btn_save_mission": Value Change {
        n90 = event-data() -> ()  [unwired: 1 in, 2 out]
        n91 = call "File Dialog"("pattern (all files)"=".mis") -> ("selected path"=w130:path, "cancelled"=w131:bool, "error out"=w132:errorcluster)  [unwired: 11 in, 1 out]
        n92 = call <vilib>:"Clear Errors.vi"("error in (no error)"=w132) -> ()  [unwired: 5 in, 2 out]
        n93 = case shown="True" w131 {
          tunnel: w130 -> [w133 _]
          frame False {
            n94 = local read "Test Mission"() -> (w134:T19[])
            n95 = Write to Binary File(file (use dialog)=w133, data=w134) -> ()  [unwired: 4 in, 3 out]
          }
          frame True {
          }
        }
      }
      event "btn_open_mission": Value Change {
        n96 = event-data() -> ()  [unwired: 1 in, 2 out]
        n97 = call "File Dialog2"("pattern (all files)"=".mis") -> ("selected path"=w136:path, "cancelled"=w135:bool, "error out"=w137:errorcluster)  [unwired: 11 in, 1 out]
        n98 = call <vilib>:"Clear Errors.vi"("error in (no error)"=w137) -> ()  [unwired: 5 in, 2 out]
        n99 = case shown="False" w135 {
          tunnel: w136 -> [w141 _]
          frame False {
            n100 = Read from Binary File(5:T19[] [] ("Test Mission"), 11:w141) -> (2:w139:T19[])  [unwired: 4 in, 3 out]
            n101 = local write "Test Mission"(w139) -> ()
          }
          frame True {
          }
        }
      }
      event "btn_set_aip_min_depth": Value Change {
        n102 = event-data() -> ()  [unwired: 1 in, 1 out]
        n103 = Get Date/Time In Seconds() -> (seconds since 1Jan1904=w148:timestamp)
        n104 = call "Write Msg Header.vi"("Sender Name"="mr. testy", "Time Stamp"=w148, "Msg ID"=RDS_Message_ID."AIP_Set_Min_Depth", "RDS Message in"=refnum<class "AIP Set Min Depth Message.lvclass"> refnum ("RDS Child Messages.lvlib:AIP Set Min Depth Message.lvclass")) -> ("RDS Message out"=w144:refnum<class "AIP Set Min Depth Message.lvclass">)  [unwired: 6 in, 1 out]
        n105 = call "Write Min Depth Message.vi"("Min Depth"="AIP Min Depth", "AIP Set Min Depth Message in"=w144) -> ("AIP Set Min Depth Message out"=w142:refnum<class "AIP Set Min Depth Message.lvclass">)  [unwired: 8 in, 1 out]
        n106 = call "RDS Child Send Msg.vi"("RDS Message"=w142, "RDS Parent Actor in"=w146) -> ()  [unwired: 8 in, 2 out]
      }
      event "btn_set_mag_dev": Value Change {
        n107 = event-data() -> ()  [unwired: 1 in, 1 out]
        n108 = call "Pack Mag Dev Msg.vi"("Compass Mag Dev"="Compass Mag Dev") -> ("Set Mag Dev Message out"=w150:refnum<class "Set Mag Dev Message.lvclass">)  [unwired: 10 in]
        n109 = call "RDS Child Send Msg.vi"("RDS Message"=w150, "RDS Parent Actor in"=w152) -> ()  [unwired: 8 in, 2 out]
      }
      event "btn_upload_mission": Value Change {
        n110 = event-data() -> ()  [unwired: 1 in, 1 out]
        n111 = call "Pack Mission Upload Message.vi"("Test Mission"="Test Mission") -> ("Mission Upload Message out"=w153:refnum<class "Mission Upload Message.lvclass">)  [unwired: 10 in]
        n112 = call "RDS Child Send Msg.vi"("RDS Message"=w153, "RDS Parent Actor in"=w155) -> ()  [unwired: 8 in, 2 out]
      }
      event "btn_set_op_run": Value Change {
        n113 = event-data() -> ()  [unwired: 1 in, 2 out]
        n114 = call "Pack SetOp And Run.vi"("MissionOp Index"="MissionOp Index") -> ("Mission Set Op Index and Run Msg out"=w156:refnum<class "Mission Set Op Index and Run Msg.lvclass">)  [unwired: 10 in]
        n115 = call "RDS Child Send Msg.vi"("RDS Message"=w156, "RDS Parent Actor in"=w157) -> ()  [unwired: 8 in, 2 out]
      }
      event "btn_send settings": Value Change {
        n116 = event-data() -> ()  [unwired: 1 in, 2 out]
        n117 = call "Pack Mission Mission Settings Message.vi"("Mission Controller Settings"="Mission Controller Settings") -> ("Set Mission Controller Settings Message out"=w159:refnum<class "Set Mission Controller Settings Message.lvclass">)  [unwired: 10 in]
        n118 = call "RDS Child Send Msg.vi"("RDS Message"=w159, "RDS Parent Actor in"=w160) -> ()  [unwired: 8 in, 2 out]
      }
      event "RDS State": Value Change {
        n119 = event-data() -> ()  [unwired: 1 in, 2 out]
        n120 = call "Read Robodolf Controller State.vi"("RDS State in"="RDS State") -> ("Controller State"=→"Controller State":T23)  [unwired: 8 in, 2 out]
        n121 = call "Read Mission Controller State.vi"("RDS State in"="RDS State") -> ("Mission Controller State"=w172:T20)  [unwired: 8 in, 2 out]
        "Mission Controller State" <- w172
        n122 = call "Read Helm Status.vi"("RDS State in"="RDS State") -> ("Helm Status"=→"Helm Status 2":T15)  [unwired: 8 in, 2 out]
        n123 = Unbundle By Name(w172) -> ("Nav State.GPS Latitude"=w168:ext, "Nav State.GPS Longitude"=w167:ext, "Mission"=w171:T19[], "Current MissionOp Index"=w170:i32)
        n124 = Index Array(array=w171, index=w170) -> (element=w169:T19)
        n125 = Bundle("GPS Latitude"=w168, "GPS Longitude"=w167) -> (w164:cluster{"GPS Latitude":ext, "GPS Longitude":ext})  [unwired: 1 in]
        n126 = Unbundle By Name(w169) -> ("GPS Latitude"=w166:dbl, "GPS Longitude"=w165:dbl)
        n127 = Bundle("GPS Latitude"=w166, "GPS Longitude"=w165) -> (w162:cluster{"GPS Latitude":dbl, "GPS Longitude":dbl})  [unwired: 1 in]
        n128 = Build Array(w164, w162) -> (→"XY Graph":T18)
      }
      event "btn_local_remote_Relinquish": Value Change {
        n129 = event-data() -> ()  [unwired: 1 in, 1 out]
        n130 = Get Date/Time In Seconds() -> (seconds since 1Jan1904=w186:timestamp)
        n131 = call "Write Msg Header.vi"("Sender Name"="mr. testy", "Time Stamp"=w186, "Msg ID"=RDS_Message_ID."Controller_Message", "RDS Message in"=refnum<class "Controller Message.lvclass"> refnum ("RDS Child Messages.lvlib:Controller Message.lvclass")) -> ("error out"=w182:errorcluster, "RDS Message out"=w181:refnum<class "Controller Message.lvclass">)  [unwired: 6 in]
        n132 = call "Write Controller Message Type.vi"("error in (no error)"=w182, "Controller Message Type"=Controller_Message_Type."Control Relinquish Request", "Controller Message in"=w181) -> ("error out"=w178:errorcluster, "Controller Message out"=w179:refnum<class "Controller Message.lvclass">)  [unwired: 7 in]
        n133 = call "Write Controller Address.vi"("error in (no error)"=w178, "Controller"=Controller."Local Remote Control", "Controller Message in"=w179) -> ("Controller Message out"=w177:refnum<class "Controller Message.lvclass">)  [unwired: 7 in, 1 out]
        n134 = call "RDS Child Send Msg.vi"("RDS Message"=w177, "RDS Parent Actor in"=w184) -> ()  [unwired: 8 in, 2 out]
      }
      event "btn_shore_remote_Relinquish": Value Change {
        n135 = event-data() -> ()  [unwired: 1 in, 1 out]
        n136 = Get Date/Time In Seconds() -> (seconds since 1Jan1904=w198:timestamp)
        n137 = call "Write Msg Header.vi"("Sender Name"="mr. testy", "Time Stamp"=w198, "Msg ID"=RDS_Message_ID."Controller_Message", "RDS Message in"=refnum<class "Controller Message.lvclass"> refnum ("RDS Child Messages.lvlib:Controller Message.lvclass")) -> ("error out"=w194:errorcluster, "RDS Message out"=w193:refnum<class "Controller Message.lvclass">)  [unwired: 6 in]
        n138 = call "Write Controller Message Type.vi"("error in (no error)"=w194, "Controller Message Type"=Controller_Message_Type."Control Relinquish Request", "Controller Message in"=w193) -> ("error out"=w190:errorcluster, "Controller Message out"=w191:refnum<class "Controller Message.lvclass">)  [unwired: 7 in]
        n139 = call "Write Controller Address.vi"("error in (no error)"=w190, "Controller"=Controller."Shore Remote Control", "Controller Message in"=w191) -> ("Controller Message out"=w189:refnum<class "Controller Message.lvclass">)  [unwired: 7 in, 1 out]
        n140 = call "RDS Child Send Msg.vi"("RDS Message"=w189, "RDS Parent Actor in"=w196) -> ()  [unwired: 8 in, 2 out]
      }
      event "btn_shore_remote_ReqControl": Value Change {
        n141 = event-data() -> ()  [unwired: 1 in, 1 out]
        n142 = Get Date/Time In Seconds() -> (seconds since 1Jan1904=w210:timestamp)
        n143 = call "Write Msg Header.vi"("Sender Name"="mr. testy", "Time Stamp"=w210, "Msg ID"=RDS_Message_ID."Controller_Message", "RDS Message in"=refnum<class "Controller Message.lvclass"> refnum ("RDS Child Messages.lvlib:Controller Message.lvclass")) -> ("error out"=w206:errorcluster, "RDS Message out"=w205:refnum<class "Controller Message.lvclass">)  [unwired: 6 in]
        n144 = call "Write Controller Message Type.vi"("error in (no error)"=w206, "Controller Message Type"=Controller_Message_Type."Control Request", "Controller Message in"=w205) -> ("error out"=w202:errorcluster, "Controller Message out"=w203:refnum<class "Controller Message.lvclass">)  [unwired: 7 in]
        n145 = call "Write Controller Address.vi"("error in (no error)"=w202, "Controller"=Controller."Shore Remote Control", "Controller Message in"=w203) -> ("Controller Message out"=w201:refnum<class "Controller Message.lvclass">)  [unwired: 7 in, 1 out]
        n146 = call "RDS Child Send Msg.vi"("RDS Message"=w201, "RDS Parent Actor in"=w208) -> ()  [unwired: 8 in, 2 out]
      }
      event "btn_mission_Relinquish": Value Change {
        n147 = event-data() -> ()  [unwired: 1 in, 1 out]
        n148 = Get Date/Time In Seconds() -> (seconds since 1Jan1904=w222:timestamp)
        n149 = call "Write Msg Header.vi"("Sender Name"="mr. testy", "Time Stamp"=w222, "Msg ID"=RDS_Message_ID."Controller_Message", "RDS Message in"=refnum<class "Controller Message.lvclass"> refnum ("RDS Child Messages.lvlib:Controller Message.lvclass")) -> ("error out"=w218:errorcluster, "RDS Message out"=w217:refnum<class "Controller Message.lvclass">)  [unwired: 6 in]
        n150 = call "Write Controller Message Type.vi"("error in (no error)"=w218, "Controller Message Type"=Controller_Message_Type."Control Relinquish Request", "Controller Message in"=w217) -> ("error out"=w214:errorcluster, "Controller Message out"=w215:refnum<class "Controller Message.lvclass">)  [unwired: 7 in]
        n151 = call "Write Controller Address.vi"("error in (no error)"=w214, "Controller"=Controller."Mission Control", "Controller Message in"=w215) -> ("Controller Message out"=w213:refnum<class "Controller Message.lvclass">)  [unwired: 7 in, 1 out]
        n152 = call "RDS Child Send Msg.vi"("RDS Message"=w213, "RDS Parent Actor in"=w220) -> ()  [unwired: 8 in, 2 out]
      }
      event "btn_mission_ReqControl": Value Change {
        n153 = event-data() -> ()  [unwired: 1 in, 1 out]
        n154 = Get Date/Time In Seconds() -> (seconds since 1Jan1904=w234:timestamp)
        n155 = call "Write Msg Header.vi"("Sender Name"="mr. testy", "Time Stamp"=w234, "Msg ID"=RDS_Message_ID."Controller_Message", "RDS Message in"=refnum<class "Controller Message.lvclass"> refnum ("RDS Child Messages.lvlib:Controller Message.lvclass")) -> ("error out"=w230:errorcluster, "RDS Message out"=w229:refnum<class "Controller Message.lvclass">)  [unwired: 6 in]
        n156 = call "Write Controller Message Type.vi"("error in (no error)"=w230, "Controller Message Type"=Controller_Message_Type."Control Request", "Controller Message in"=w229) -> ("error out"=w226:errorcluster, "Controller Message out"=w227:refnum<class "Controller Message.lvclass">)  [unwired: 7 in]
        n157 = call "Write Controller Address.vi"("error in (no error)"=w226, "Controller"=Controller."Mission Control", "Controller Message in"=w227) -> ("Controller Message out"=w225:refnum<class "Controller Message.lvclass">)  [unwired: 7 in, 1 out]
        n158 = call "RDS Child Send Msg.vi"("RDS Message"=w225, "RDS Parent Actor in"=w232) -> ()  [unwired: 8 in, 2 out]
      }
      event "Port Motor Time": Value Change {
        n159 = event-data() -> ("NewVal"=w238:timestamp)  [unwired: 1 in, 1 out]
        n160 = Get Date/Time In Seconds() -> (seconds since 1Jan1904=w237:timestamp)
        n161 = Subtract(x=w237, y=w238) -> (x-y=→"Message time":dbl)
      }
      event "Btn STBD Throttle": Value Change {
        n162 = event-data() -> ()  [unwired: 1 in, 1 out]
        n163 = Get Date/Time In Seconds() -> (seconds since 1Jan1904=w246:timestamp)
        n164 = call "Write Msg Header.vi"("Sender Name"="mr. testy", "Time Stamp"=w246, "Msg ID"=RDS_Message_ID."MCB_Command", "RDS Message in"=refnum<class "MCB Command.lvclass"> refnum ("RDS Child Messages.lvlib:MCB Command.lvclass")) -> ("RDS Message out"=w242:refnum<class "MCB Command.lvclass">)  [unwired: 6 in, 1 out]
        n165 = call "Write Motor Command.vi"("Motor Command"="STBD Throttle", "Motor"=MCB_Channel."STBD", "MCB Command in"=w242) -> ("MCB Command out"=w240:refnum<class "MCB Command.lvclass">)  [unwired: 7 in, 1 out]
        n166 = call "RDS Child Send Msg.vi"("RDS Message"=w240, "RDS Parent Actor in"=w244) -> ()  [unwired: 8 in, 2 out]
      }
      event "AIP Stow": Value Change {
        n167 = event-data() -> ()  [unwired: 1 in, 1 out]
        n168 = Get Date/Time In Seconds() -> (seconds since 1Jan1904=w252:timestamp)
        n169 = call "Write Msg Header.vi"("Sender Name"="mr. testy", "Time Stamp"=w252, "Msg ID"=RDS_Message_ID."AIP_Command", "RDS Message in"=refnum<class "AIP Command.lvclass"> refnum ("RDS Child Messages.lvlib:AIP Command.lvclass")) -> ("RDS Message out"=w253:refnum<class "AIP Command.lvclass">)  [unwired: 6 in, 1 out]
        n170 = call "Write AIP.vi"("AIP Command"=AIP_Command_Control."Stow", "AIP Deploy Command in"=w253) -> ("AIP Deploy Command out"=w249:refnum<class "AIP Command.lvclass">)  [unwired: 8 in, 1 out]
        n171 = call "RDS Child Send Msg.vi"("RDS Message"=w249, "RDS Parent Actor in"=w248) -> ()  [unwired: 8 in, 2 out]
      }
      event "AIP Stop": Value Change {
        n172 = event-data() -> ()  [unwired: 1 in, 1 out]
        n173 = Get Date/Time In Seconds() -> (seconds since 1Jan1904=w260:timestamp)
        n174 = call "Write Msg Header.vi"("Sender Name"="mr. testy", "Time Stamp"=w260, "Msg ID"=RDS_Message_ID."AIP_Command", "RDS Message in"=refnum<class "AIP Command.lvclass"> refnum ("RDS Child Messages.lvlib:AIP Command.lvclass")) -> ("RDS Message out"=w261:refnum<class "AIP Command.lvclass">)  [unwired: 6 in, 1 out]
        n175 = call "Write AIP.vi"("AIP Command"=AIP_Command_Control."Stop", "AIP Deploy Command in"=w261) -> ("AIP Deploy Command out"=w257:refnum<class "AIP Command.lvclass">)  [unwired: 8 in, 1 out]
        n176 = call "RDS Child Send Msg.vi"("RDS Message"=w257, "RDS Parent Actor in"=w256) -> ()  [unwired: 8 in, 2 out]
      }
      event "btn_shutdown": Value Change {
        n177 = event-data() -> ()  [unwired: 1 in, 1 out]
        n178 = Two Button Dialog(message="WARNING!\n\nAre you sure you want to shutdown the battery?\n\nSystem will cut power in 60 seconds if you click yes ") -> (T button?=w264:bool)  [unwired: 2 in]
        n179 = case shown="True" w264 {
          tunnel: w266 -> [_ w268]
          frame False {
          }
          frame True {
            n180 = Get Date/Time In Seconds() -> (seconds since 1Jan1904=w270:timestamp)
            n181 = call "Write Msg Header.vi"("Sender Name"="mr. testy", "Time Stamp"=w270, "Msg ID"=RDS_Message_ID."BTB_Shutdown") -> ("RDS Message out"=w267:refnum<class "RDS Message.lvclass">)  [unwired: 7 in, 1 out]
            n182 = call "RDS Child Send Msg.vi"("RDS Message"=w267, "RDS Parent Actor in"=w268) -> ()  [unwired: 8 in, 2 out]
          }
        }
      }
      event "Send string": Value Change {
        n183 = event-data() -> ()  [unwired: 1 in, 1 out]
        n184 = call "Write Msg Header.vi"("Sender Name"="Cock", "Msg ID"=RDS_Message_ID."String Message", "RDS Message in"=refnum<class "String Message.lvclass"> refnum ("RDS Child Messages.lvlib:String Message.lvclass")) -> ("RDS Message out"=w275:refnum<class "String Message.lvclass">)  [unwired: 7 in, 1 out]
        n185 = call "Write String.vi"("String"="String 2", "String Message in"=w275) -> ("String Message out"=w272:refnum<class "String Message.lvclass">)  [unwired: 8 in, 1 out]
        n186 = call "RDS Child Send Msg.vi"("RDS Message"=w272, "RDS Parent Actor in"=w278) -> ()  [unwired: 8 in, 2 out]
      }
    }
  }
  n187 = call-parent "Actor Core.vi"("error in"=w33, "Actor in"=w29) -> ("error out"=→"error out":errorcluster, "Actor out"=→"Actor out":refnum<class "Actor.lvclass">)  [unwired: 8 in]
